vi "Verify VI.vi"(7 "Test VI (caller)":string, 8 "error in":errorcluster, 10 "VI to Verify":path) -> (0 "error out":errorcluster)   [LabVIEW 2020, in "Caraya.Extension.lvlib"]
uses:
  Caraya.Extension.lvlib
  <vilib>/addons/_JKI Toolkits/Caraya/classes/Assert/Assert True.vi
  <vilib>/addons/_JKI Toolkits/Caraya/classes/Assert/Assert.lvclass
  Approval Tests/Approval Tests.lvlib
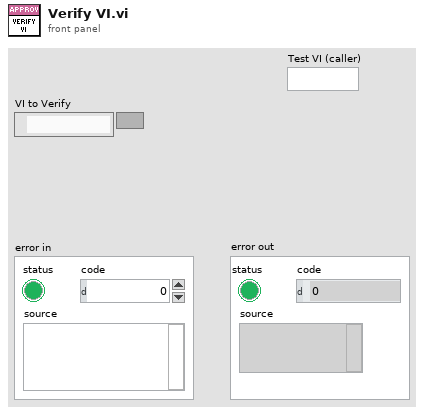
[diagram p1: front panel]
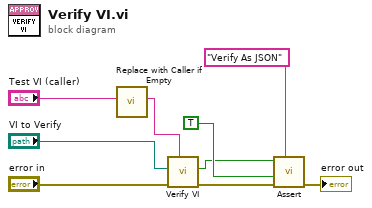
[diagram p0: block diagram]
diagram:
  n1 = call "Replace with Caller if Empty.vi"("Test VI (caller) in"="Test VI (caller)") -> ("Test VI (caller) out"=w1:string)  [unwired: 10 in]
  n2 = call "Verify VI.vi"("Test VI (caller)"=w1, "error in"="error in", "Path to VI to Verify"="VI to Verify") -> ("error out"=w5:errorcluster, "Passed?"=w4:bool)  [unwired: 6 in, 1 out]
  n3 = call-poly <vilib>:"Assert.vi"("Label"="Verify As JSON", "error in (no error)"=w5, "Register with caller test (F)"=TRUE, "True?"=w4) -> ("error out"=→"error out":errorcluster)  [unwired: 6 in, 1 out]
